vi "PicoScope4000aGetStreamingValues.vi"(10 "handle in":i16, 11 "error in":errorcluster) -> (0 "Start Index in Driver Buffer":u32, 1 "Trigger":cluster{bool, "triggeredAt (Total samples)":u32}, 2 "handle out":i16, 3 "error out":errorcluster, 4 "Number of Samples":u32, 5 "ready":i16, 6 "Auto Stopped":bool)   [LabVIEW 2016]
doc: "This VI is used in streaming mode to get the latest values from the driver. It should be called in a loop after the oscilloscope has been set up using PicoScope3000aSettings.vi and streaming has been started by calling PicoScope3000aStartStreaming.vi. The VI outputs the number of samples available and the start index of these samples in the array output by PicoScope3000aStartStreaming.vi."
uses:
  ps4000aWrap.dll
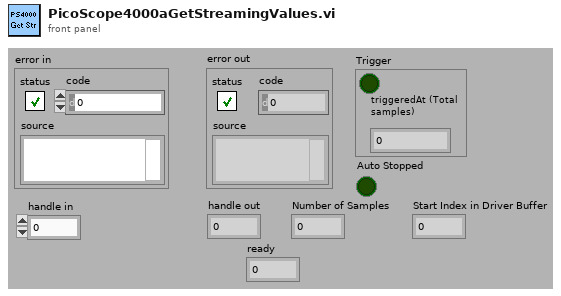
[diagram p1: front panel]
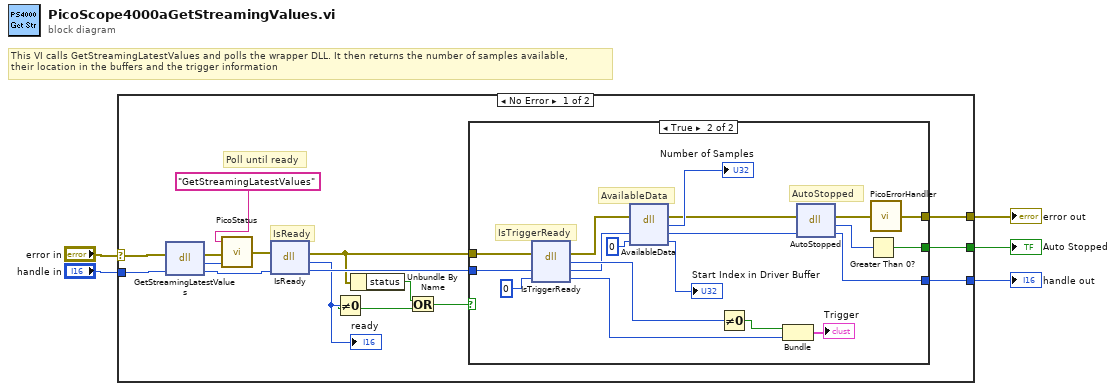
[diagram p0: block diagram]
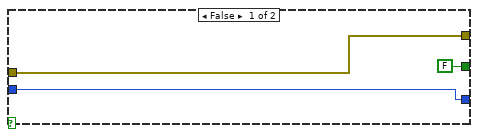
[diagram p2: hidden frame]
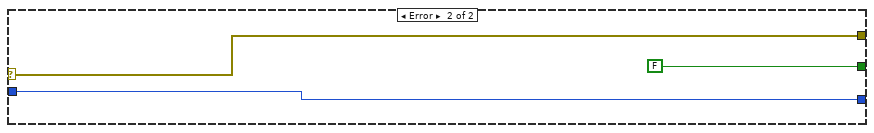
[diagram p3: hidden frame]
diagram:
  # "This VI calls GetStreamingLatestValues and polls the wrapper DLL. It then returns the number of samples available, \ntheir location in the buffers and the trigger information"
  n1 = case shown="No Error" "error in" {
    selector: "error in" -> [w16 w46]
    tunnel: [w21 w46] -> w4
    tunnel: "handle in" -> [w15 w45]
    tunnel: [w18 w45] -> w2
    tunnel: [w17 FALSE] -> w1
    frame No Error {
      # "IsReady"
      # "Poll until ready"
      n2 = dll-call lib="ps4000aWrap.dll" fn="GetStreamingLatestValues" ("PS5000.dll:_ps5000SetDataBuffer@16")(error in=w16, "handle"=w15) -> (error out=w10:errorcluster, "PICO_STATUS"=w11:u32, "handle"=w9:i16)  [unwired: 2 in, 1 out]
      n3 = call "PicoStatus.vi"("PICO STATUS"=w11, "error in"=w10, "source"="GetStreamingLatestValues") -> ("error out"=w8:errorcluster)
      n4 = dll-call lib="ps4000aWrap.dll" fn="IsReady" ("PS5000.dll:_ps5000SetDataBuffer@16")(error in=w8, "handle"=w9) -> (error out=w19:errorcluster, "ready"=w14:i16, "handle"=w20:i16)  [unwired: 2 in, 1 out]
      "ready" <- w14
      n5 = Not Equal To 0?(x=w14) -> (x != 0?=w12:bool)
      n6 = Unbundle By Name(w19) -> ("status"=w13:bool)
      n7 = Or(x=w13, y=w12) -> (x .or. y?=w6:bool)
      n8 = case shown="True" w6 {
        tunnel: [w23 w43] -> w21
        tunnel: w20 -> [w22 w41]
        tunnel: w19 -> [w23 w33]
        tunnel: [w22 w29] -> w18
        tunnel: [FALSE w27] -> w17
        frame False {
        }
        frame True {
          # "AutoStopped"
          # "AvailableData"
          # "IsTriggerReady"
          n9 = dll-call lib="ps4000aWrap.dll" fn="IsTriggerReady" ("PS5000.dll:_ps5000SetDataBuffer@16")(error in=w33, "handle"=w41, "triggeredAt"=u32 0) -> (error out=w37:errorcluster, "triggered"=w40:i16, "handle"=w36:i16, "triggeredAt"=w25:u32)  [unwired: 2 in, 1 out]
          n10 = dll-call lib="ps4000aWrap.dll" fn="AvailableData" ("PS5000.dll:_ps5000Stop@4")(error in=w37, "handle"=w36, "startIndex"=u32 0) -> (error out=w32:errorcluster, "numSamples"=→"Number of Samples":u32, "handle"=w30:i16, "startIndex"=→"Start Index in Driver Buffer":u32)  [unwired: 2 in, 1 out]
          n11 = Not Equal To 0?(x=w40) -> (x != 0?=w39:bool)
          n12 = Bundle(w39, "triggeredAt"=w25) -> (→"Trigger":cluster{bool, "triggeredAt":u32})  [unwired: 1 in]
          n13 = dll-call lib="ps4000aWrap.dll" fn="AutoStopped"(error in=w32, "handle"=w30) -> (error out=w31:errorcluster, "autoStopped"=w28:i16, "handle"=w29:i16)  [unwired: 2 in, 1 out]
          n14 = Greater Than 0?(x=w28) -> (x > 0?=w27:bool)
          n15 = call "PicoErrorHandler.vi"("error in"=w31) -> ("error out"=w43:errorcluster)
        }
      }
    }
    frame Error {
    }
  }
  "error out" <- w4
  "handle out" <- w2
  "Auto Stopped" <- w1
